vi "Create_folders_for_SPIM_storage.vi"(10 "Prefix for image filenames":string, 11 "File Path to save DCIMG files":path) -> (1 "Arm1 path":path, 2 "SpimA path":path, 3 "SpimB path":path, 4 "Arm2 path":path)   [LabVIEW 2016]
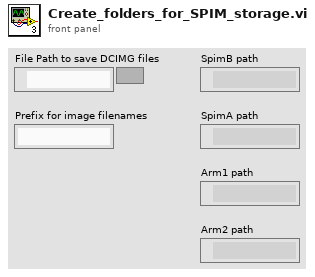
[diagram p1: front panel]
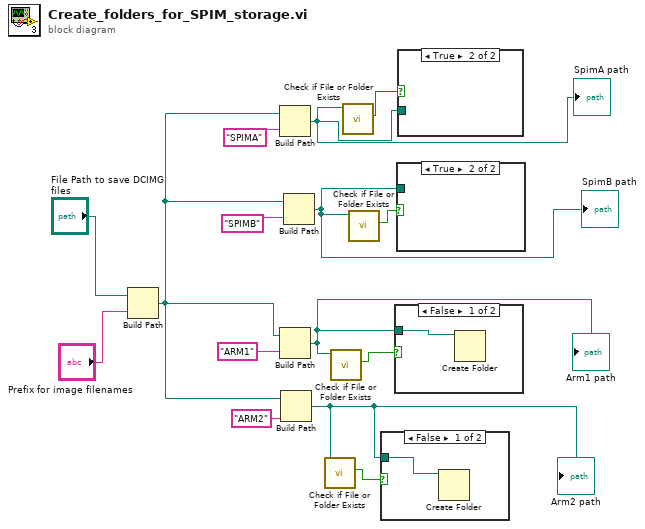
[diagram p0: block diagram]
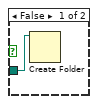
[diagram p4: hidden frame]
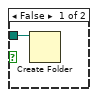
[diagram p5: hidden frame]
diagram:
  n1 = Build Path(base path="File Path to save DCIMG files", name or relative path="Prefix for image filenames") -> (appended path=w14:path)
  n2 = Build Path(base path=w14, name or relative path="SPIMA") -> (appended path=w15:path)
  "SpimA path" <- w15
  n3 = Build Path(base path=w14, name or relative path="ARM1") -> (appended path=w13:path)
  "Arm1 path" <- w13
  n4 = Build Path(base path=w14, name or relative path="ARM2") -> (appended path=w12:path)
  "Arm2 path" <- w12
  n5 = Build Path(base path=w14, name or relative path="SPIMB") -> (appended path=w5:path)
  "SpimB path" <- w5
  n6 = call <vilib>:"Check if File or Folder Exists.vi"("path"=w12) -> ("file or folder exists?"=w11:bool)  [unwired: 8 in, 2 out]
  n7 = call <vilib>:"Check if File or Folder Exists.vi"("path"=w13) -> ("file or folder exists?"=w10:bool)  [unwired: 8 in, 2 out]
  n8 = call <vilib>:"Check if File or Folder Exists.vi"("path"=w15) -> ("file or folder exists?"=w2:bool)  [unwired: 8 in, 2 out]
  n9 = call <vilib>:"Check if File or Folder Exists.vi"("path"=w5) -> ("file or folder exists?"=w1:bool)  [unwired: 8 in, 2 out]
  n10 = case shown="False" w11 {
    tunnel: w12 -> [w16 _]
    frame False {
      n11 = Create Folder(path (use dialog)=w16) -> ()  [unwired: 2 in, 3 out]
    }
    frame True {
    }
  }
  n12 = case shown="False" w10 {
    tunnel: w13 -> [w17 _]
    frame False {
      n13 = Create Folder(path (use dialog)=w17) -> ()  [unwired: 2 in, 3 out]
    }
    frame True {
    }
  }
  n14 = case shown="True" w1 {
    tunnel: w5 -> [w18 _]
    frame False {
      n15 = Create Folder(path (use dialog)=w18) -> ()  [unwired: 2 in, 3 out]
    }
    frame True {
    }
  }
  n16 = case shown="True" w2 {
    tunnel: w15 -> [w19 _]
    frame False {
      n17 = Create Folder(path (use dialog)=w19) -> ()  [unwired: 2 in, 3 out]
    }
    frame True {
    }
  }
